vi "Can_Tipper.vi"(10 "Can_Tip_Flip":bool, 11 "Can_Tip_Arm":bool) -> (2 "Can_Tip_Flip":bool, 3 "Can_Tip_Arm":bool)   [LabVIEW 2014]
panel:
  in  "Time_Flipper_On":i32=500
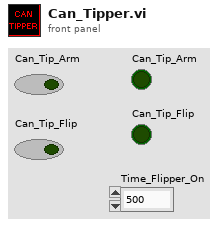
[diagram p1: front panel]
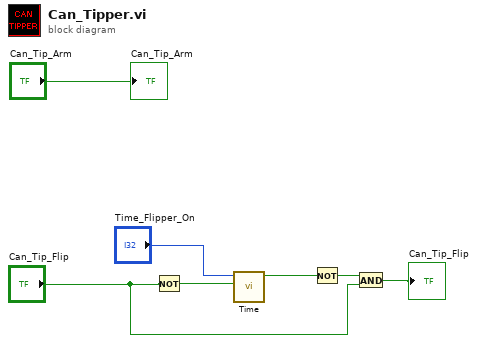
[diagram p0: block diagram]
diagram:
  n1 = Not(x="Can_Tip_Flip") -> (.not. x?=w6:bool)
  n2 = call "Time.vi"("Reset"=w6, "Time_Limit"="Time_Flipper_On") -> ("Time_Met"=w5:bool)  [unwired: 9 in]
  n3 = Not(x=w5) -> (.not. x?=w4:bool)
  n4 = And(x=w4, y="Can_Tip_Flip") -> (x .and. y?=→"Can_Tip_Flip":bool)
  "Can_Tip_Arm" <- "Can_Tip_Arm"
